vi "IV.vi"() -> ()   [LabVIEW 2018]
uses:
  support/Message Queue/Kapitza Message Queue.lvlib
  support/User Event - Stop/Kapitza User Event - Stop.lvlib
  Classes/Abstract/Experiment/Experiment2D/Experiment2D.lvclass
  support/Message Queue/Enqueue Message (Single).vi
  <vilib>/ErrorRing/Error Ring.xnode
  <vilib>/Utility/error.llb/Error Cluster From Error Code.vi
  Classes/Abstract/Measurement/Measurement2D/Measurement2D.lvclass
  Classes/Abstract/Data/Data2D/Data2D.lvclass
  Classes/2D/IV/meas/IV_meas.lvclass
  Classes/Abstract/Instrument/Instrument/Instrument.lvclass
panel:
  in  "Stop":bool
  in  "Sample Name":string
  in  "Max":dbl
  in  "Step":dbl
  in  "Init":dbl
  in  "x0,5 step":bool
  out "y":dbl
  out "x":dbl
  in  "x2 step":bool
  out "XY Graph":cluster{"X":dbl[], "Y":dbl[]}[](graph)
  in  "Start":bool
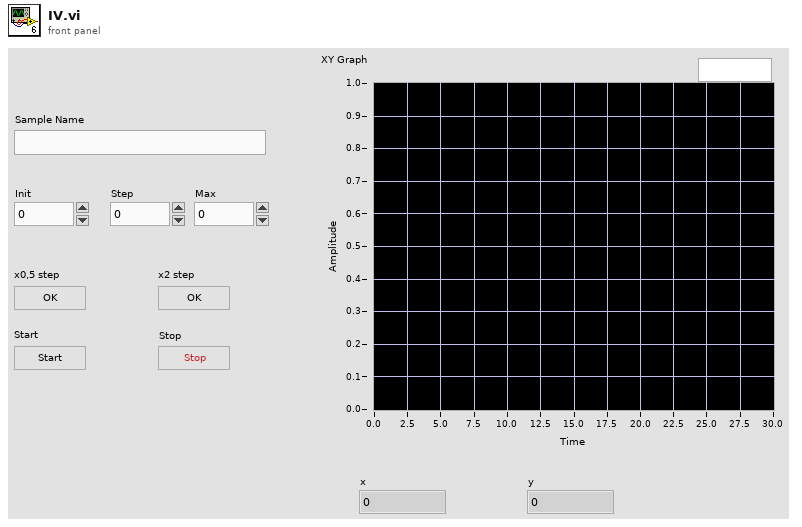
[diagram p1: front panel]
types:
  T1 = typedef "Kapitza Message Queue.lvlib/All Message Queues.ctl" = cluster{"UI":refnum<queue>}
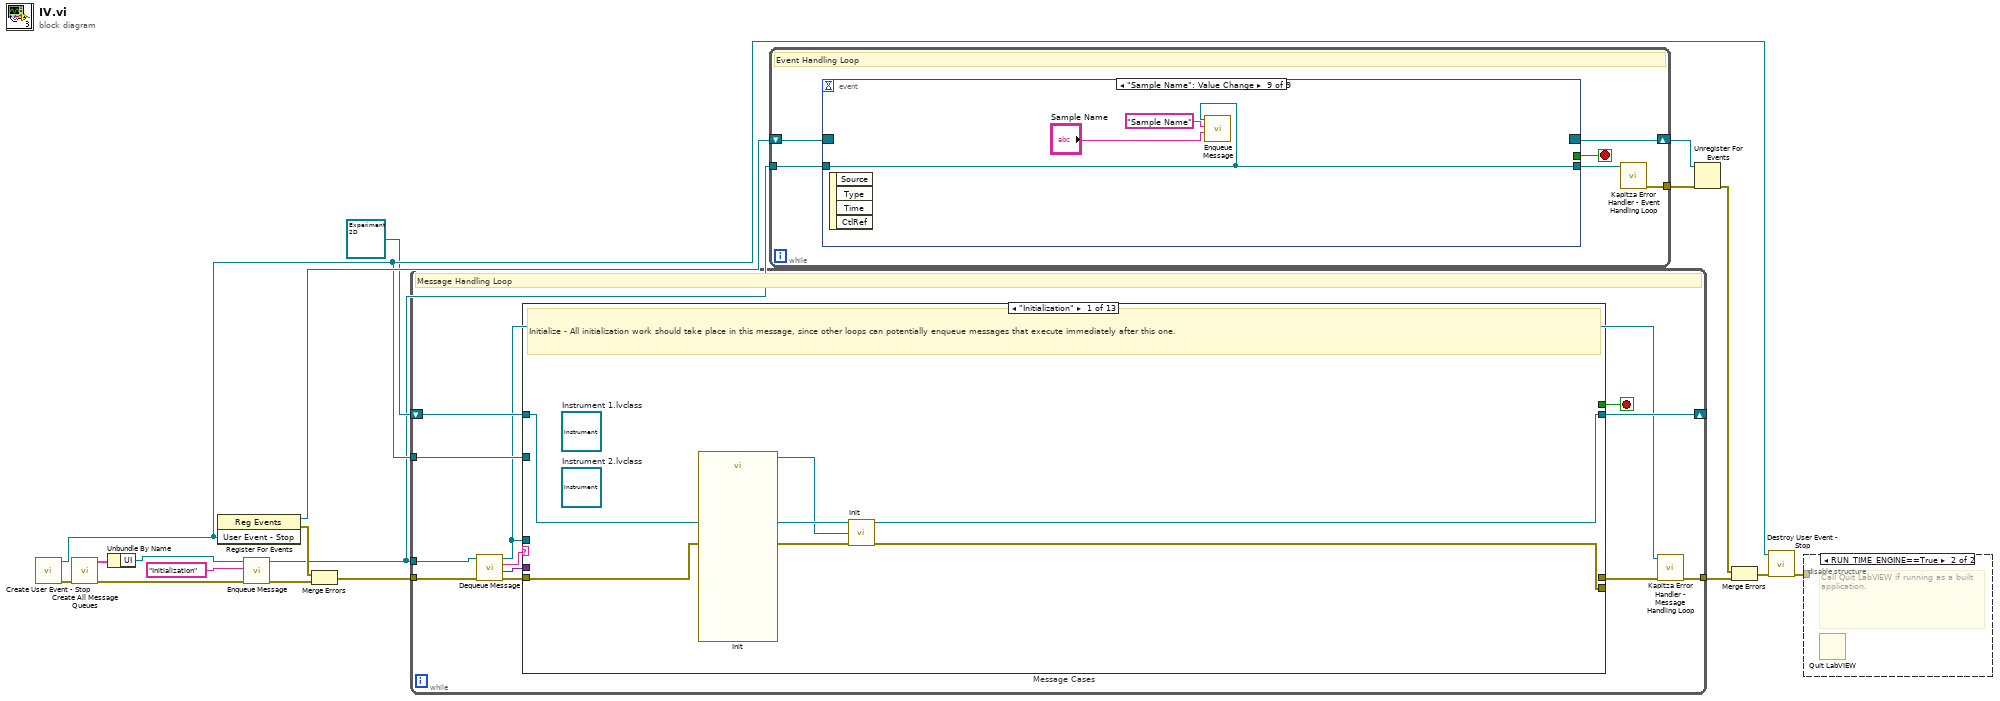
[diagram p0: block diagram]
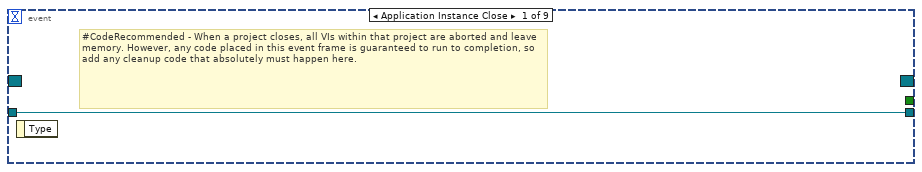
[diagram p3: hidden frame]
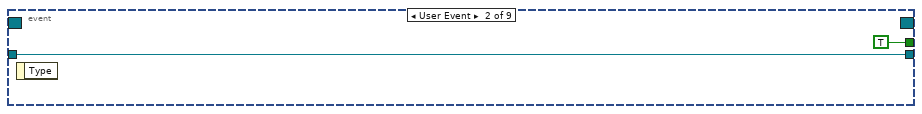
[diagram p4: hidden frame]
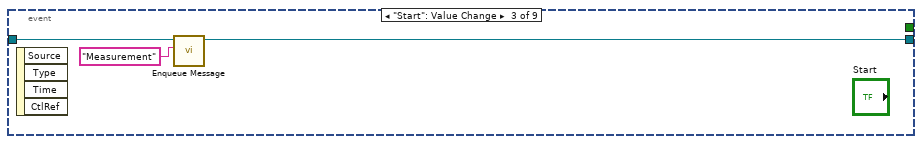
[diagram p5: hidden frame]
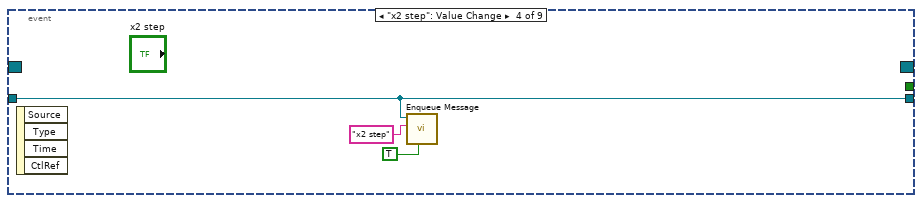
[diagram p6: hidden frame]
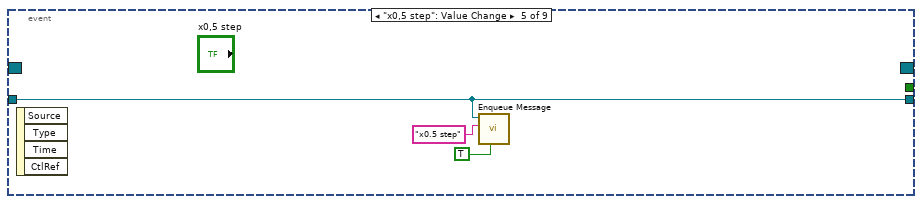
[diagram p7: hidden frame]
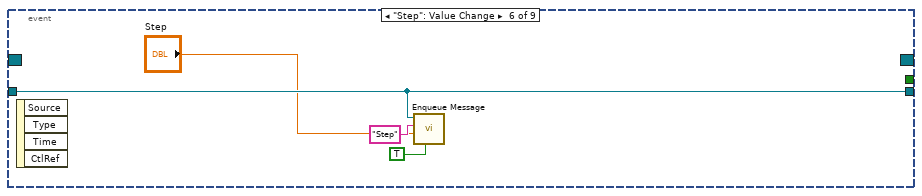
[diagram p8: hidden frame]
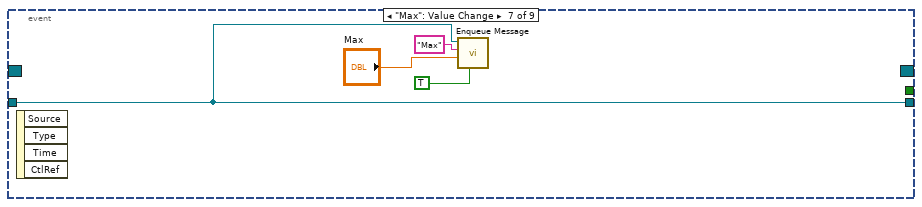
[diagram p9: hidden frame]
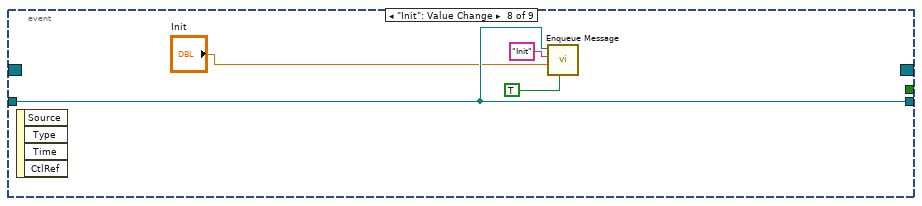
[diagram p10: hidden frame]
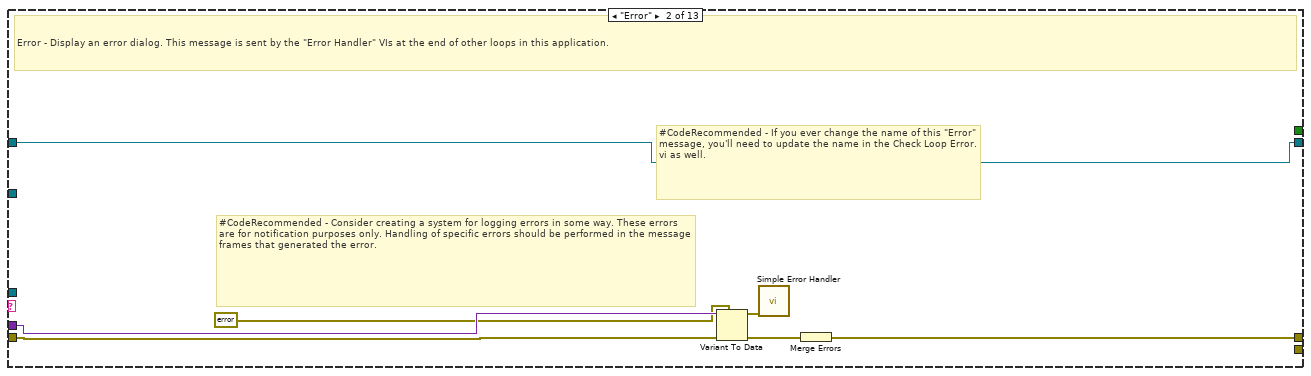
[diagram p11: hidden frame]
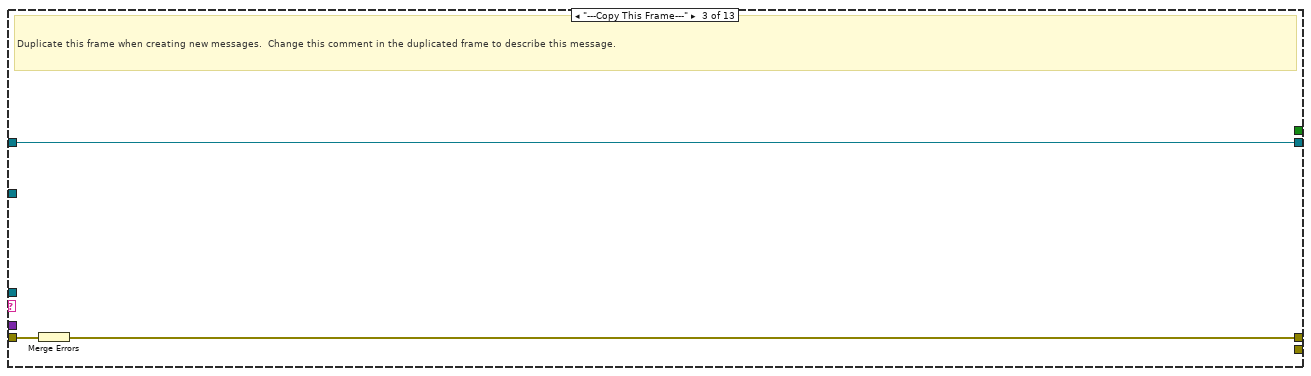
[diagram p12: hidden frame]
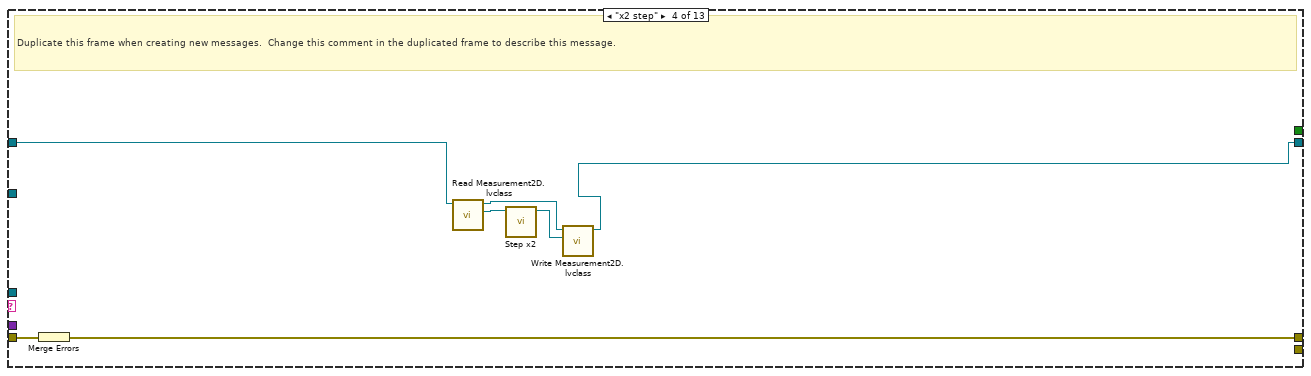
[diagram p13: hidden frame]
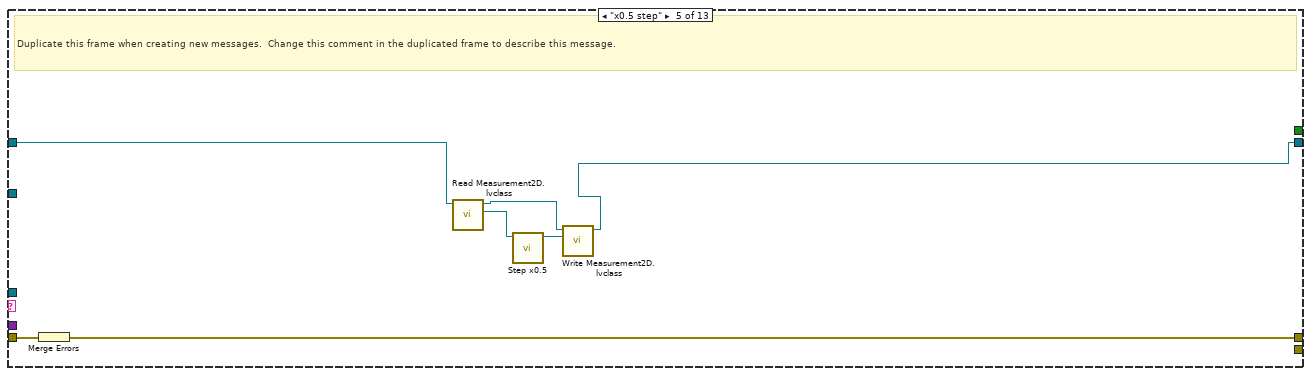
[diagram p14: hidden frame]
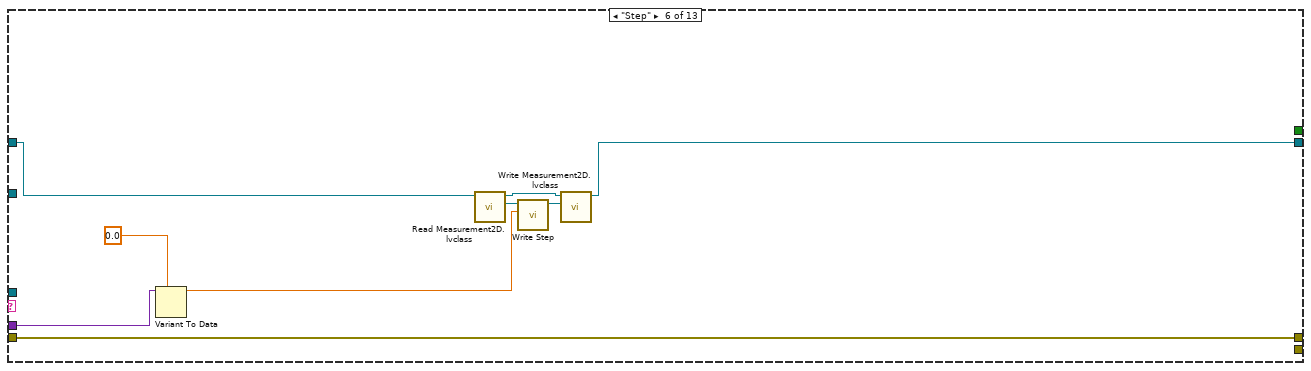
[diagram p15: hidden frame]
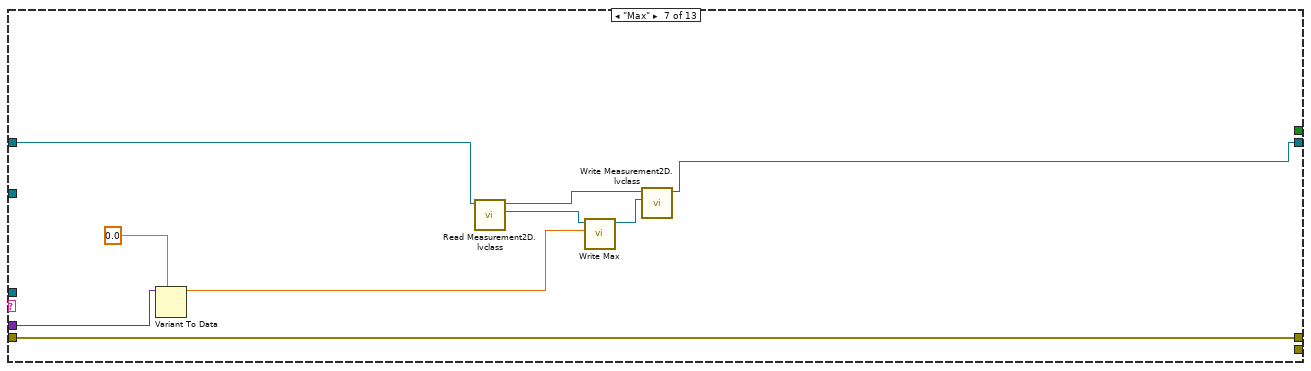
[diagram p16: hidden frame]
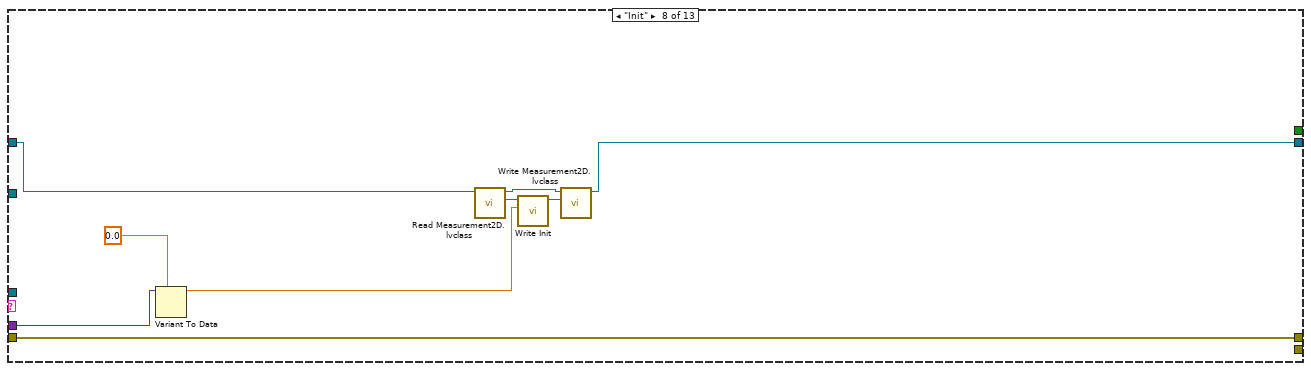
[diagram p17: hidden frame]
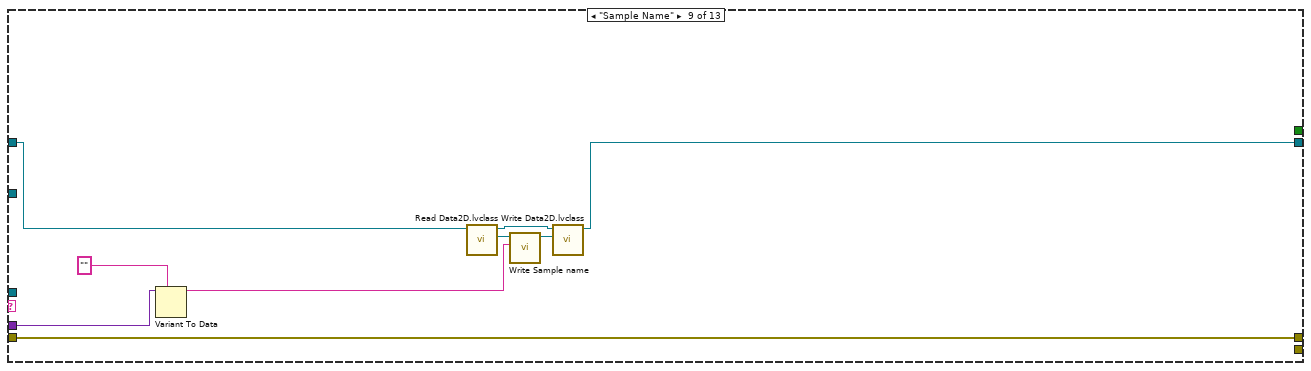
[diagram p18: hidden frame]
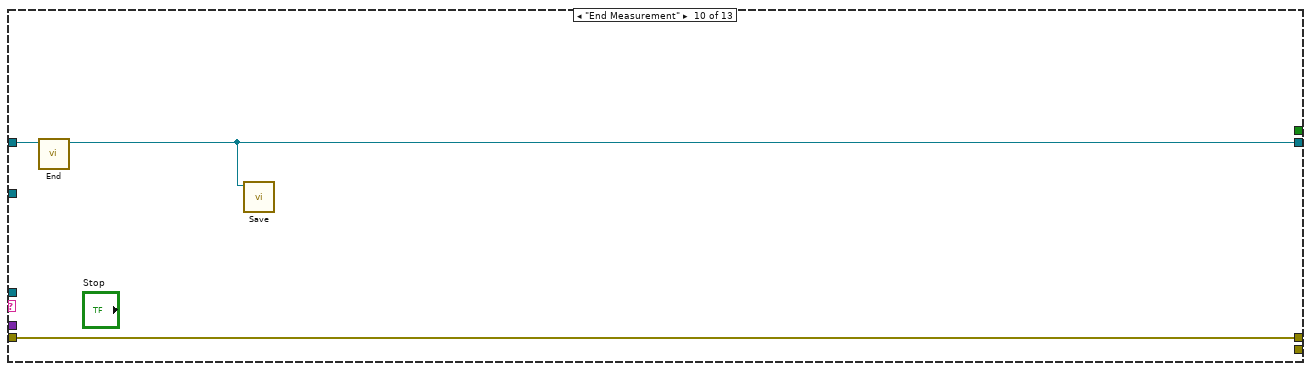
[diagram p19: hidden frame]
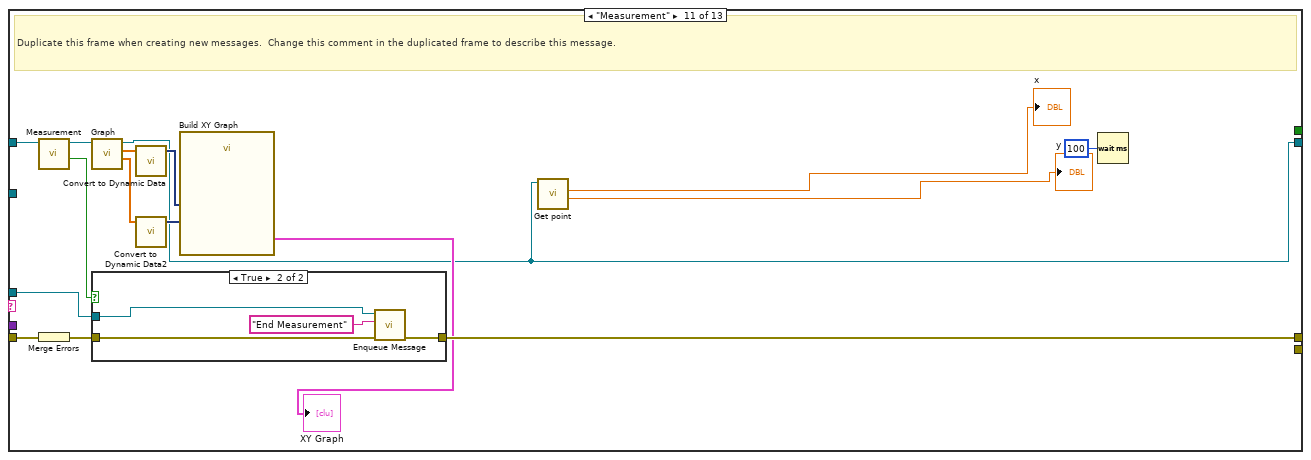
[diagram p20: hidden frame]
diagram:
  n1 = call "Create User Event - Stop.vi"() -> ("error out"=w16:errorcluster, "User Event - Stop"=w9:refnum<user-event>)  [unwired: 10 in]
  n2 = call "Create All Message Queues.vi"("error in (no error)"=w16) -> ("error out"=w1:errorcluster, "Message Queues out"=w18:T1)  [unwired: 9 in]
  n3 = Unbundle By Name(w18) -> ("UI"=w4:refnum<queue>)
  n4 = register-events(w9) -> (reference out=w10:refnum<event-registration>, error out=w7:errorcluster)  [unwired: 2 in]
  n5 = call-poly "Enqueue Message.vi"("error in (no error)"=w1, "Message"="Initialization", "Message Queue"=w4) -> ("error out"=w2:errorcluster, "dup Message Queue"=w5:refnum<queue>)  [unwired: 7 in]
  n6 = Merge Errors(w7, w2) -> (w8:errorcluster)
  n7 = while {
    tunnel: w5 -> [w22]
    shift-right: [w29] -> _
    shift-left: refnum<class "Experiment2D.lvclass"> refnum ("Experiment2D.lvclass") -> [w30]
    tunnel: w9 -> [w27]
    tunnel: w8 -> [w26]
    tunnel: [w20] -> w17
    stop <- w28 stop-if-true
    # "Message Handling Loop"
    n8 = call "Dequeue Message.vi"("error in (no error)"=w26, "Message Queue"=w22) -> ("error out"=w25:errorcluster, "Message Data"=w23:variant, "Message"=w24:string, "dup Message Queue"=w21:refnum<queue>)  [unwired: 6 in]
    n9 = case "Message Cases" shown="\"Initialization\"" w24 {
      selector: w24 -> [_ _ _ _ _ _ _ _ _ _ _ _ w134]
      tunnel: w21 -> [_ _ _ _ _ _ _ _ _ _ w111 w133 _]
      tunnel: w25 -> [w34 w42 w45 w52 w59 w68 w77 w86 w95 w98 w114 w126 _]
      tunnel: [_ w36 w43 w51 w58 w68 w77 w86 w95 w98 w109 w129 w135] -> w19
      tunnel: w30 -> [w35 w41 w44 w50 w57 w64 w70 w82 w92 w97 w113 w132 w136]
      tunnel: [w33 w41 w44 w46 w55 w63 w69 w81 w91 w96 w101 w132 w136] -> w29
      tunnel: [_ _ _ _ _ _ _ _ _ _ _ TRUE _] -> w28
      tunnel: w23 -> [_ w40 _ _ _ w67 w76 w85 w94 _ _ w123 _]
      tunnel: w27 -> [_ _ _ _ _ _ _ _ _ _ _ w128 _]
      tunnel: [w32 _ _ _ _ _ _ _ _ _ _ _ _] -> _
      frame "Initialization" {
        (unwired) refnum<class "Instrument.lvclass"> refnum  # Instrument 2.lvclass
        (unwired) refnum<class "Instrument.lvclass"> refnum  # Instrument 1.lvclass
        # "Initialize - All initialization work should take place in this message, since other loops can potentially enqueue messages that execute immediately after this one."
        n10 = call-dynamic "Init.vi"() -> ("Measurement1D out"=w31:refnum<class "IV_meas.lvclass">)  [unwired: 10 in, 1 out]
        n11 = call-dynamic "Init.vi"("Experiment2D in"=w35, "Measurement2D.lvclass"=w31, "error in (no error)"=w34) -> ("Experiment2D out"=w33:refnum<class "Experiment2D.lvclass">, "error out"=w32:errorcluster)  [unwired: 11 in]
      }
      frame "Error" {
        # "#CodeRecommended - If you ever change the name of this \"Error\" message, you'll need to update the name in the Check Loop Error.vi as well."
        # "#CodeRecommended - Consider creating a system for logging errors in some way. These errors are for notification purposes only. Handling of specific errors should be performed in the message frames that generated the error."
        # "Error - Display an error dialog. This message is sent by the \"Error Handler\" VIs at the end of other loops in this application."
        n12 = Variant To Data(error in=w42, type=errorcluster {"status"=FALSE, "code"=0, "source"=""} ("error constant"), Variant=w40) -> (data=w38:errorcluster, error out=w37:errorcluster)
        n13 = call <vilib>:"Simple Error Handler.vi"("error in (no error)"=w38) -> ()  [unwired: 4 in, 5 out]
        n14 = Merge Errors(w37) -> (w36:errorcluster)
      }
      frame "---Copy This Frame---" {
        # "Duplicate this frame when creating new messages.  Change this comment in the duplicated frame to describe this message."
        n15 = Merge Errors(w45) -> (w43:errorcluster)
      }
      frame "x2 step" {
        # "Duplicate this frame when creating new messages.  Change this comment in the duplicated frame to describe this message."
        n16 = Merge Errors(w52) -> (w51:errorcluster)
        n17 = call-dynamic "Read Measurement2D.lvclass.vi"("Experiment2D in"=w50) -> ("Measurement2D.lvclass"=w49:refnum<class "Measurement2D.lvclass">, "Experiment2D out"=w48:refnum<class "Experiment2D.lvclass">)  [unwired: 8 in, 1 out]
        n18 = call-dynamic "Step x2.vi"("Measurement2D in"=w49) -> ("Measurement2D out"=w47:refnum<class "Measurement2D.lvclass">)  [unwired: 9 in, 1 out]
        n19 = call-dynamic "Write Measurement2D.lvclass.vi"("Measurement2D.lvclass"=w47, "Experiment2D in"=w48) -> ("Experiment2D out"=w46:refnum<class "Experiment2D.lvclass">)  [unwired: 8 in, 1 out]
      }
      frame "x0.5 step" {
        # "Duplicate this frame when creating new messages.  Change this comment in the duplicated frame to describe this message."
        n20 = Merge Errors(w59) -> (w58:errorcluster)
        n21 = call-dynamic "Read Measurement2D.lvclass.vi"("Experiment2D in"=w57) -> ("Measurement2D.lvclass"=w54:refnum<class "Measurement2D.lvclass">, "Experiment2D out"=w56:refnum<class "Experiment2D.lvclass">)  [unwired: 8 in, 1 out]
        n22 = call-dynamic "Step x0.5.vi"("Measurement2D in"=w54) -> ("Measurement2D out"=w53:refnum<class "Measurement2D.lvclass">)  [unwired: 9 in, 1 out]
        n23 = call-dynamic "Write Measurement2D.lvclass.vi"("Measurement2D.lvclass"=w53, "Experiment2D in"=w56) -> ("Experiment2D out"=w55:refnum<class "Experiment2D.lvclass">)  [unwired: 8 in, 1 out]
      }
      frame "Step" {
        n24 = Variant To Data(type=0.0, Variant=w67) -> (data=w61:dbl)  [unwired: 1 in, 1 out]
        n25 = call-dynamic "Read Measurement2D.lvclass.vi"("Experiment2D in"=w64) -> ("Measurement2D.lvclass"=w62:refnum<class "Measurement2D.lvclass">, "Experiment2D out"=w65:refnum<class "Experiment2D.lvclass">)  [unwired: 8 in, 1 out]
        n26 = call-dynamic "Write Step.vi"("Step"=w61, "Measurement2D in"=w62) -> ("Measurement2D out"=w60:refnum<class "Measurement2D.lvclass">)  [unwired: 8 in, 1 out]
        n27 = call-dynamic "Write Measurement2D.lvclass.vi"("Measurement2D.lvclass"=w60, "Experiment2D in"=w65) -> ("Experiment2D out"=w63:refnum<class "Experiment2D.lvclass">)  [unwired: 8 in, 1 out]
      }
      frame "Max" {
        n28 = Variant To Data(type=0.0, Variant=w76) -> (data=w74:dbl)  [unwired: 1 in, 1 out]
        n29 = call-dynamic "Read Measurement2D.lvclass.vi"("Experiment2D in"=w70) -> ("Measurement2D.lvclass"=w73:refnum<class "Measurement2D.lvclass">, "Experiment2D out"=w71:refnum<class "Experiment2D.lvclass">)  [unwired: 8 in, 1 out]
        n30 = call-dynamic "Write Max.vi"("Max"=w74, "Measurement2D in"=w73) -> ("Measurement2D out"=w72:refnum<class "Measurement2D.lvclass">)  [unwired: 8 in, 1 out]
        n31 = call-dynamic "Write Measurement2D.lvclass.vi"("Measurement2D.lvclass"=w72, "Experiment2D in"=w71) -> ("Experiment2D out"=w69:refnum<class "Experiment2D.lvclass">)  [unwired: 8 in, 1 out]
      }
      frame "Init" {
        n32 = Variant To Data(type=0.0, Variant=w85) -> (data=w79:dbl)  [unwired: 1 in, 1 out]
        n33 = call-dynamic "Read Measurement2D.lvclass.vi"("Experiment2D in"=w82) -> ("Measurement2D.lvclass"=w80:refnum<class "Measurement2D.lvclass">, "Experiment2D out"=w83:refnum<class "Experiment2D.lvclass">)  [unwired: 8 in, 1 out]
        n34 = call-dynamic "Write Init.vi"("Init"=w79, "Measurement2D in"=w80) -> ("Measurement2D out"=w78:refnum<class "Measurement2D.lvclass">)  [unwired: 8 in, 1 out]
        n35 = call-dynamic "Write Measurement2D.lvclass.vi"("Measurement2D.lvclass"=w78, "Experiment2D in"=w83) -> ("Experiment2D out"=w81:refnum<class "Experiment2D.lvclass">)  [unwired: 8 in, 1 out]
      }
      frame "Sample Name" {
        n36 = Variant To Data(type="", Variant=w94) -> (data=w90:string)  [unwired: 1 in, 1 out]
        n37 = call-dynamic "Read Data2D.lvclass.vi"("Experiment2D in"=w92) -> ("Data2D.lvclass"=w89:refnum<class "Data2D.lvclass">, "Experiment2D out"=w87:refnum<class "Experiment2D.lvclass">)  [unwired: 8 in, 1 out]
        n38 = call-dynamic "Write Sample name.vi"("Sample name"=w90, "Data2D in"=w89) -> ("Data2D out"=w88:refnum<class "Data2D.lvclass">)  [unwired: 8 in, 1 out]
        n39 = call-dynamic "Write Data2D.lvclass.vi"("Data2D.lvclass"=w88, "Experiment2D in"=w87) -> ("Experiment2D out"=w91:refnum<class "Experiment2D.lvclass">)  [unwired: 8 in, 1 out]
      }
      frame "End Measurement" {
        n40 = call-dynamic "End.vi"("Experiment2D in"=w97) -> ("Experiment2D out"=w96:refnum<class "Experiment2D.lvclass">)  [unwired: 9 in, 1 out]
        n41 = call-dynamic "Save.vi"("Experiment2D in"=w96) -> ()  [unwired: 9 in, 2 out]
      }
      frame "Measurement" {
        # "Duplicate this frame when creating new messages.  Change this comment in the duplicated frame to describe this message."
        n42 = call-dynamic "Measurement.vi"("Experiment2D in"=w113) -> ("Finish?"=w112:bool, "Experiment2D out"=w108:refnum<class "Experiment2D.lvclass">)  [unwired: 7 in, 2 out]
        n43 = Merge Errors(w114) -> (w110:errorcluster)
        n44 = call-dynamic "Graph.vi"("Experiment2D in"=w108) -> ("Y"=w102:dbl[], "X"=w103:dbl[], "Experiment2D out"=w101:refnum<class "Experiment2D.lvclass">)  [unwired: 7 in, 1 out]
        n45 = case shown="True" w112 {
          tunnel: w111 -> [w117 w122]
          tunnel: w110 -> [w116 w120]
          tunnel: [w115 w119] -> w109
          frame False {
            n46 = call-poly "Enqueue Message.vi"("error in (no error)"=w116, "Message"="Measurement", "Message Queue"=w117) -> ("error out"=w115:errorcluster)  [unwired: 7 in, 1 out]
          }
          frame True {
            n47 = call-poly "Enqueue Message.vi"("error in (no error)"=w120, "Message"="End Measurement", "Message Queue"=w122) -> ("error out"=w119:errorcluster)  [unwired: 7 in, 1 out]
          }
        }
        n48 = call "Convert to Dynamic Data"("Array"=w103) -> ("Dynamic Data Type"=w106:dynamicdata)  [unwired: 3 in]
        n49 = call "Convert to Dynamic Data2"("Array"=w102) -> ("Dynamic Data Type"=w105:dynamicdata)  [unwired: 3 in]
        n50 = call "Build XY Graph"("Y Input"=w105, "X Input"=w106) -> ("XY Graph"=→"XY Graph":cluster{"X":dbl[], "Y":dbl[]}[])  [unwired: 8 in, 1 out]
        n51 = call-dynamic "Get point.vi"("Experiment2D in"=w101) -> ("y"=→"y":dbl, "x"=→"x":dbl)  [unwired: 7 in, 2 out]
        n52 = Wait (ms)(milliseconds to wait=u32 100) -> ()  [unwired: 1 out]
      }
      frame "Exit" {
        # "Stop the VI"
        # "Release the message queue reference"
        # "#CodeNeeded - Add any required cleanup code here. Note that if 'Exit' was called as a result of an error, an error dialog will be displayed. Add any custom error handling for an 'Exit' condition here as well."
        # "Exit - Exit the application."
        n53 = call "Fire User Event - Stop.vi"("User Event - Stop"=w128) -> ("error out"=w127:errorcluster)  [unwired: 10 in]
        n54 = Release Queue(queue=w133, error in (no error)=w126) -> (error out=w130:errorcluster)  [unwired: 1 in, 2 out]
        n55 = Variant To Data(type=errorcluster {"status"=FALSE, "code"=0, "source"=""} ("error constant"), Variant=w123) -> (data=w124:errorcluster)  [unwired: 1 in, 1 out]
        n56 = Merge Errors(w127, w130) -> (w129:errorcluster)
        n57 = call <vilib>:"Simple Error Handler.vi"("error in (no error)"=w124) -> ()  [unwired: 4 in, 5 out]
      }
      frame Default {
        # "'Default' case only runs if there is a message that isn't defined in any of the other cases.  Output a programming error."
        n58 = disable-structure shown="Enabled" {
          disable-tunnel: [w138 _] -> w135
          disable-tunnel: w134 -> [w137 _]
          frame Disabled {
            n59 = xnode "Error Ring"("parameter 0"=w137) -> ("error out"=w138:errorcluster)
          }
          frame Enabled {
          }
        }
      }
    }
    n60 = call "Kapitza Error Handler - Message Handling Loop.vi"("error in (no error)"=w19, "Message Queue"=w21) -> ("dup error in"=w20:errorcluster)  [unwired: 8 in, 1 out]
  }
  n61 = while {
    tunnel: w5 -> [w151]
    shift-right: [w149] -> w13
    shift-left: w10 -> [w150]
    tunnel: [w146] -> w11
    stop <- w148 stop-if-true
    # "Event Handling Loop"
    n62 = event shown="[8] \"Sample Name\": Value Change" {
      selector: w150 -> [_ _ _ _ _ _ _ _ _]
      dyn-events: [_ _ _ _ _ _ _ _ _] -> w149
      timeout: _ -> [_ _ _ _ _ _ _ _ _]
      tunnel: [_ TRUE ("Discard?") _ _ _ _ _ _ _] -> w148
      tunnel: w151 -> [w152 w154 w157 w160 w161 w166 w169 w173 w177]
      tunnel: [w152 w154 w156 w160 w161 w166 w169 w173 w177] -> w147
      event Application Instance Close {
        # "#CodeRecommended - When a project closes, all VIs within that project are aborted and leave memory. However, any code placed in this event frame is guaranteed to run to completion, so add any cleanup code that absolutely must happen here."
        n63 = event-data() -> ()  [unwired: 1 in, 1 out]
      }
      event User Event {
        n64 = event-data() -> ()  [unwired: 1 in, 1 out]
      }
      event "Start": Value Change {
        n65 = event-data() -> ()  [unwired: 1 in, 4 out]
        n66 = call-poly "Enqueue Message.vi"("Message"="Measurement", "Message Queue"=w157) -> ("dup Message Queue"=w156:refnum<queue>)  [unwired: 8 in, 1 out]
      }
      event "x2 step": Value Change {
        n67 = event-data() -> ()  [unwired: 1 in, 4 out]
        n68 = call-poly "Enqueue Message.vi"("Priority Message? (F)"=TRUE, "Message"="x2 step", "Message Queue"=w160) -> ()  [unwired: 7 in, 2 out]
      }
      event "x0,5 step": Value Change {
        n69 = event-data() -> ()  [unwired: 1 in, 4 out]
        n70 = call-poly "Enqueue Message.vi"("Priority Message? (F)"=TRUE, "Message"="x0.5 step", "Message Queue"=w161) -> ()  [unwired: 7 in, 2 out]
      }
      event "Step": Value Change {
        n71 = event-data() -> ()  [unwired: 1 in, 4 out]
        n72 = call-poly "Enqueue Message.vi"("Priority Message? (F)"=TRUE, "Message Data"="Step", "Message"="Step", "Message Queue"=w166) -> ()  [unwired: 6 in, 2 out]
      }
      event "Max": Value Change {
        n73 = event-data() -> ()  [unwired: 1 in, 4 out]
        n74 = call-poly "Enqueue Message.vi"("Priority Message? (F)"=TRUE, "Message Data"="Max", "Message"="Max", "Message Queue"=w169) -> ()  [unwired: 6 in, 2 out]
      }
      event "Init": Value Change {
        n75 = event-data() -> ()  [unwired: 1 in, 4 out]
        n76 = call-poly "Enqueue Message.vi"("Priority Message? (F)"=TRUE, "Message Data"="Init", "Message"="Init", "Message Queue"=w173) -> ()  [unwired: 6 in, 2 out]
      }
      event "Sample Name": Value Change {
        n77 = event-data() -> ()  [unwired: 1 in, 4 out]
        n78 = call-poly "Enqueue Message.vi"("Message Data"="Sample Name", "Message"="Sample Name", "Message Queue"=w177) -> ()  [unwired: 7 in, 2 out]
      }
    }
    n79 = call "Kapitza Error Handler - Event Handling Loop.vi"("Message Queue"=w147) -> ("dup error in"=w146:errorcluster)  [unwired: 9 in, 1 out]
  }
  n80 = Unregister For Events(event registration refnum=w13, error in=w11) -> (error out=w14:errorcluster)
  n81 = Merge Errors(w14, w17) -> (w15:errorcluster)
  n82 = call "Destroy User Event - Stop.vi"("error in (no error)"=w15, "User Event - Stop"=w9) -> ("error out"=w12:errorcluster)  [unwired: 9 in]
  n83 = disable-structure shown="RUN_TIME_ENGINE==True" {
    disable-tunnel: w12 -> [_ _]
    frame condition #0 (active) {
    }
    frame condition #1 {
      # "Call Quit LabVIEW if running as a built application."
      n84 = Quit LabVIEW() -> ()  [unwired: 1 in]
    }
  }
